vi "Add Read Section.vi"(8 "error in (no error)":errorcluster, 11 "TreeControl in":refnum<vi>) -> (0 "error out":errorcluster, 2 "Read Tag":string, 3 "TreeControl out":refnum<vi>)   [LabVIEW 2012, in "Shared Variable Custom Device.lvlib"]
uses:
  Shared Variable Custom Device.lvlib
  Shared/Shared Variable Globals.vi
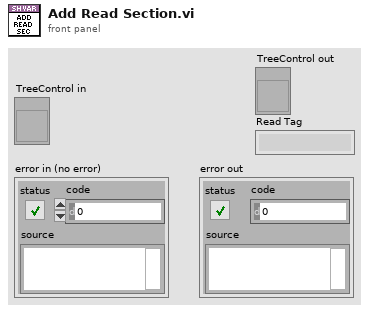
[diagram p1: front panel]
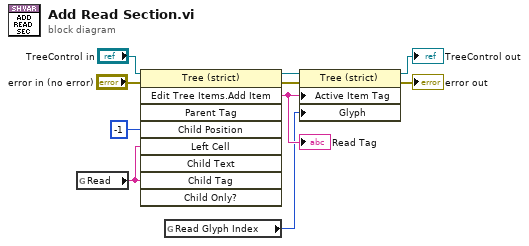
[diagram p0: block diagram]
diagram:
  n1 = global read "Shared Variable Globals.vi" "Read"() -> (w9:string)
  n2 = invoke on="Invoke Node" class="Tree (strict)" method="Edit Tree Items.Add Item"(reference="TreeControl in", error in="error in (no error)", "Child Position"=-1, "Left Cell"=w9, "Child Tag"=w9) -> (reference out=w4:refnum<vi>, error out=w5:errorcluster, "Edit Tree Items:Add Item"=w7:string)  [unwired: 4 in, 6 out]
  "Read Tag" <- w7
  n3 = global read "Shared Variable Globals.vi" "Read Glyph Index"() -> (w6:i32)
  n4 = property on="Property Node" class="Tree (strict)"(reference=w4, error in=w5, "Active Item Tag"=w7, "Glyph"=w6) -> (reference out=→"TreeControl out":refnum<vi>, error out=→"error out":errorcluster)
